vi "Get Computer Info.vi"(2 "error in (no error)":errorcluster) -> (0 "error out":errorcluster, 1 "Computer Info":string[][](table))   [LabVIEW 2016, in "Control Experiment SM.lvclass"]
uses:
  Control Experiment SM.lvclass
  System.Management
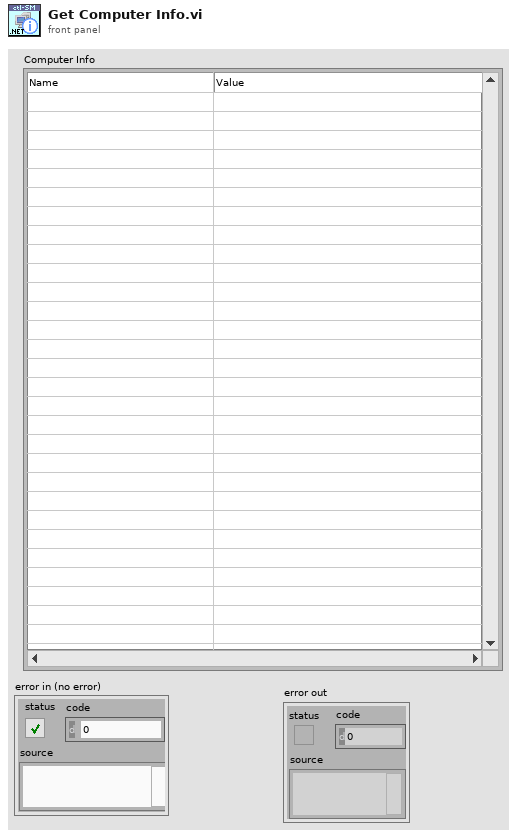
[diagram p1: front panel]
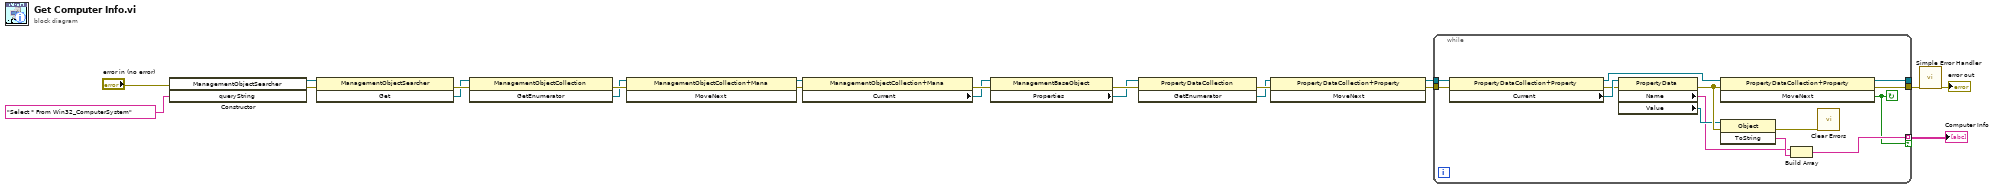
[diagram p0: block diagram]
diagram:
  n1 = constructor class="ManagementObjectSearcher"(error in="error in (no error)", "queryString"="Select * From Win32_ComputerSystem" ("query")) -> (reference out=w19:refnum<k24>, error out=w18:errorcluster)  [unwired: 2 in, 2 out]
  n2 = invoke class="ManagementObjectSearcher" method="Get"(reference=w19, error in=w18) -> (error out=w20:errorcluster, "Get"=w5:refnum<k24>)  [unwired: 1 in, 1 out]
  n3 = invoke class="ManagementObjectCollection" method="GetEnumerator"(reference=w5, error in=w20) -> (error out=w21:errorcluster, "GetEnumerator"=w4:refnum<k24>)  [unwired: 1 in, 1 out]
  n4 = invoke class="ManagementObjectCollection+Mana" method="MoveNext"(reference=w4, error in=w21) -> (reference out=w17:refnum<k24>, error out=w16:errorcluster)  [unwired: 1 in, 1 out]
  n5 = property class="ManagementObjectCollection+Mana"(reference=w17, error in=w16) -> (error out=w10:errorcluster, "Current"=w3:refnum<k24>)  [unwired: 1 out]
  n6 = property class="ManagementBaseObject"(reference=w3, error in=w10) -> (error out=w13:errorcluster, "Properties"=w2:refnum<k24>)  [unwired: 1 out]
  n7 = invoke class="PropertyDataCollection" method="GetEnumerator"(reference=w2, error in=w13) -> (error out=w14:errorcluster, "GetEnumerator"=w1:refnum<k24>)  [unwired: 1 in, 1 out]
  n8 = invoke class="PropertyDataCollection+Property" method="MoveNext"(reference=w1, error in=w14) -> (reference out=w12:refnum<k24>, error out=w15:errorcluster)  [unwired: 1 in, 1 out]
  n9 = while {
    tunnel: w12 -> [w35]
    tunnel: w15 -> [w33]
    tunnel: [w31] -> w9
    tunnel: [w30] -> _
    tunnel: [w29] -> w11 mode=indexing if=w28
    stop <- w28 continue-if-true
    n10 = property class="PropertyDataCollection+Property"(reference=w35, error in=w33) -> (reference out=w25:refnum<k24>, error out=w32:errorcluster, "Current"=w34:refnum<k24>)
    n11 = property class="PropertyData"(reference=w34, error in=w32) -> (error out=w27:errorcluster, "Name"=w22:string, "Value"=w23:refnum<k24>)  [unwired: 1 out]
    n12 = invoke class="PropertyDataCollection+Property" method="MoveNext"(reference=w25, error in=w27) -> (reference out=w30:refnum<k24>, error out=w31:errorcluster, "MoveNext"=w28:bool)  [unwired: 1 in]
    n13 = invoke class="Object" method="ToString"(reference=w23, error in=w27) -> (error out=w26:errorcluster, "ToString"=w24:string)  [unwired: 1 in, 1 out]
    n14 = Build Array(w22, w24) -> (w29:string[])
    n15 = call <vilib>:"Clear Errors.vi"("error in (no error)"=w26) -> ()  [unwired: 5 in, 2 out]
  }
  "Computer Info" <- w11
  n16 = call <vilib>:"Simple Error Handler.vi"("error in (no error)"=w9) -> ("error out"=→"error out":errorcluster)  [unwired: 4 in, 4 out]
